vi "Array_Over_Threshold (SubVI).vi"(10 "Threshold":dbl, 11 "Start Array":dbl[](array[numeric])) -> (3 "Array":dbl[](array[numeric]))   [LabVIEW 2020]
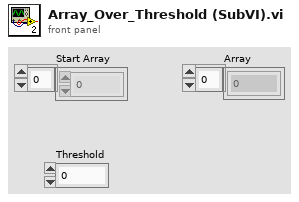
[diagram p1: front panel]
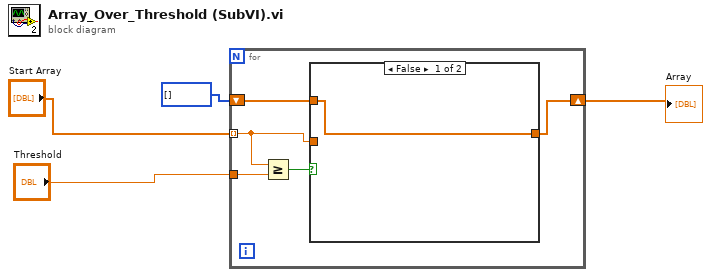
[diagram p0: block diagram]
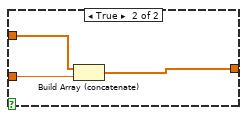
[diagram p2: hidden frame]
diagram:
  n1 = for {
    tunnel: "Threshold" -> [w8]
    tunnel: "Start Array" -> [w6] mode=indexing
    shift-right: [w5] -> w4
    shift-left: i32[] [] -> [w7]
    n2 = Greater Or Equal?(x=w6, y=w8) -> (x >= y?=w9:bool)
    n3 = case shown="False" w9 {
      tunnel: [w10 w13] -> w5
      tunnel: w7 -> [w10 w12]
      tunnel: w6 -> [_ w11]
      frame False {
      }
      frame True {
        n4 = Build Array (concatenate)(w12, w11) -> (w13:dbl[])
      }
    }
  }
  "Array" <- w4
